vi "Configure.vi"() -> (0 "Error Out":u8)   [LabVIEW 2024]
uses:
  <vilib>/rvi/eio/common/nirviEmuTemplateMethod_errors.vi
  <vilib>/rvi/Emulation/niFpgaEmulationIsFPGAContextNoSignature.vi
  <vilib>/rvi/DataTransferAndStorage/Container/Common/niFpgaContainerGetUniqueNameForEmu.vi
  <vilib>/rvi/Memory/Memory_Emulation/niFpgaMemoryEmulationCacheClearOnFirstRun.vi
  <vilib>/rvi/Memory/Memory_Emulation/nirvimemoryEmulationManagerCache_MakeExclusive.vi
  <vilib>/rvi/Memory/Memory_Emulation/niFpgaMemoryEmulationValidateCache.vi
  <vilib>/rvi/Memory/Memory_Emulation/nirvimemoryEmulationManagerCache_InsertValue.vi
  <vilib>/Utility/error.llb/Clear Errors.vi
  <vilib>/rvi/Memory/Memory_Emulation/nirvimemoryEmulationManagerCache_ReleaseExclusive.vi
  <vilib>/rvi/Memory/Memory_Emulation/nirvimemoryEmulationManagerCache_GetValue.vi
  <vilib>/rvi/Memory/Memory_Emulation/nirvimemoryEmulationManagerCache_SetValue.vi
  <vilib>/rvi/Emulation/niFpgaProcessEmulError.vi
  <vilib>/rvi/Emulation/niFpgaSctlEmulationGetInTimedLoop.vi
  <vilib>/eio/EIONode/EIONode.xnode
  <vilib>/rvi/DataTransferAndStorage/Container/XNode/niFpgaContainer.xnode
  <vilib>/rvi/DataTransferAndStorage/Register/Emulation/niFpgaRegisterEmulation.vi
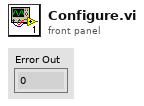
[diagram p1: front panel]
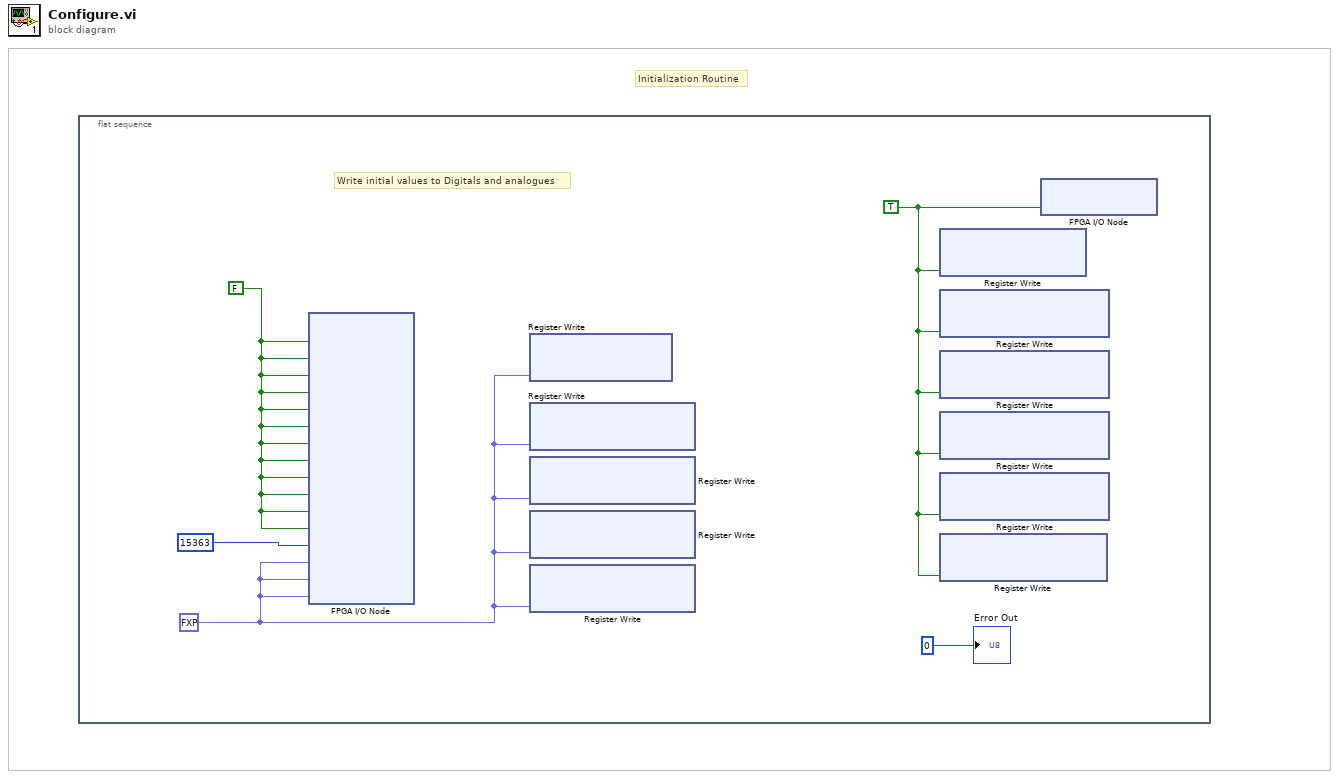
[diagram p0: block diagram]
diagram:
  # "Initialization Routine"
  n1 = flat-sequence {
    frame #0 {
      w4 = TRUE ("Interlock Out")
      w1 = fxp<+/-,20,5> 0.0 ("Mod1/AO0")
      w5 = FALSE ("Mod2/DIO0")
      # "Write initial values to Digitals and analogues"
      n2 = xnode "FPGA I/O Node"("Mod2/DIO0"=w5, "Mod2/DIO1"=w5, "Mod2/DIO2"=w5, "Mod2/DIO3"=w5, "Mod3/DIO0"=w5, "Mod3/DIO1"=w5, "Mod3/DIO2"=w5, "Mod3/DIO3"=w5, "Mod4/DIO0"=w5, "Mod4/DIO1"=w5, "Mod4/DIO2"=w5, "Mod4/DIO3"=w5, "Z Stage"=i16 15363, "Mod1/AO1"=w1, "Mod1/AO2"=w1, "Mod1/AO3"=w1) -> ()  [unwired: 16 in, 16 out]
      n3 = xnode ("Register Write")("Data"=w1) -> ()  [unwired: 1 in, 1 out]
      n4 = xnode ("Register Write")("Data"=w1) -> ()  [unwired: 1 in, 1 out]
      n5 = xnode ("Register Write")("Data"=w1) -> ()  [unwired: 1 in, 1 out]
      n6 = xnode ("Register Write")("Data"=w1) -> ()  [unwired: 1 in, 1 out]
      n7 = xnode ("Register Write")("Data"=w1) -> ()  [unwired: 1 in, 1 out]
      n8 = xnode ("Register Write")("Data"=w4) -> ()  [unwired: 1 in, 1 out]
      n9 = xnode ("Register Write")("Data"=w4) -> ()  [unwired: 1 in, 1 out]
      n10 = xnode ("Register Write")("Data"=w4) -> ()  [unwired: 1 in, 1 out]
      n11 = xnode ("Register Write")("Data"=w4) -> ()  [unwired: 1 in, 1 out]
      n12 = xnode ("Register Write")("Data"=w4) -> ()  [unwired: 1 in, 1 out]
      n13 = xnode ("Register Write")("Data"=w4) -> ()  [unwired: 1 in, 1 out]
      n14 = xnode "FPGA I/O Node"("Interlock OUT"=w4) -> ()  [unwired: 1 in, 1 out]
      "Error Out" <- u8 0 ("Error code")
    }
  }
